vi "AMC_OpenCloseConn.vi"(7 "Open":bool, 8 "error in":errorcluster, 9 "deviceAddress":string="192.168.0.3", 10 "Retry":bool, 11 "ConnID":refnum<k5>) -> (0 "error out":errorcluster, 3 "connection ID":refnum<k5>)   [LabVIEW 2019]
uses:
  <vilib>/Utility/config.llb/Read Key (U32).vi
  <vilib>/Utility/config.llb/Write Key (U32).vi
  <vilib>/Utility/config.llb/Read Key (String).vi
  <vilib>/Utility/config.llb/Read Key (I32).vi
  <vilib>/Utility/config.llb/Read Key (Boolean).vi
  <vilib>/Utility/config.llb/Write Key (String).vi
  <vilib>/Utility/config.llb/Write Key (Boolean).vi
  <vilib>/Utility/config.llb/Write Key (I32).vi
  <vilib>/Utility/config.llb/NI_LVConfig.lvlib
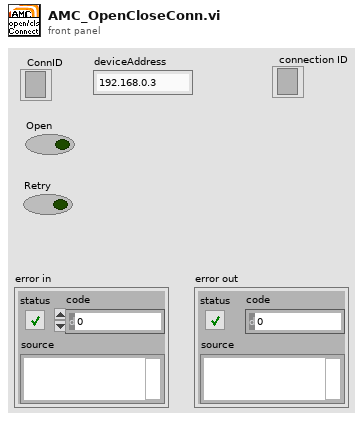
[diagram p1: front panel]
types:
  T1 = enum16{"Répertoire du VI actuel", "Répertoire du parent 1", "Répertoire du parent 2", "Répertoire du parent 3"}
  T2 = typedef "NI_LVConfig.lvlib/Config Data RefNum.ctl" = refnum<k1>
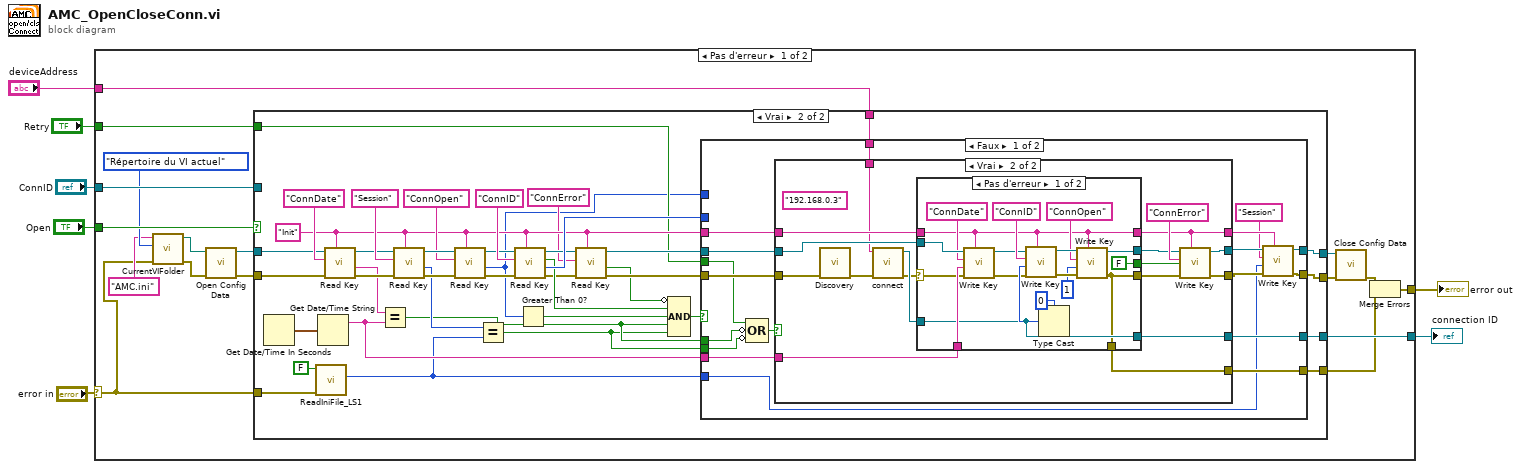
[diagram p0: block diagram]
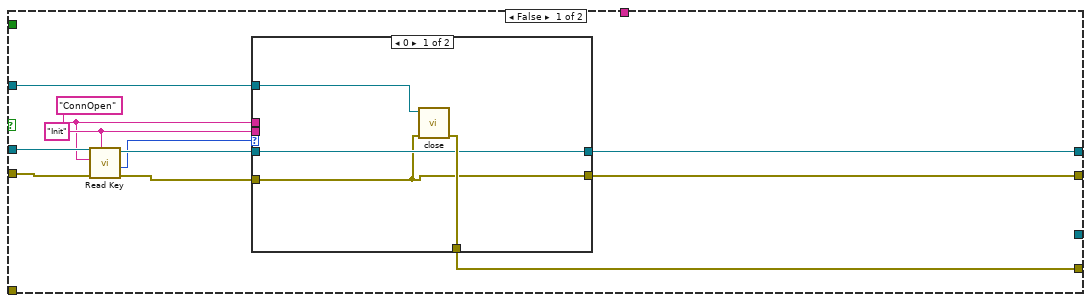
[diagram p2: hidden frame]
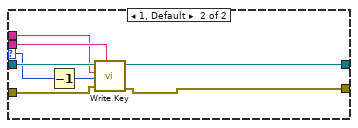
[diagram p3: hidden frame]
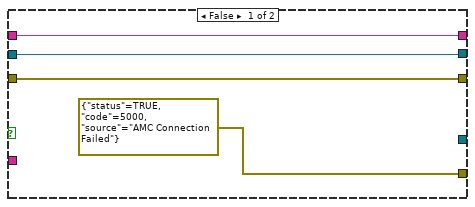
[diagram p4: hidden frame]
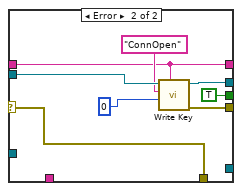
[diagram p5: hidden frame]
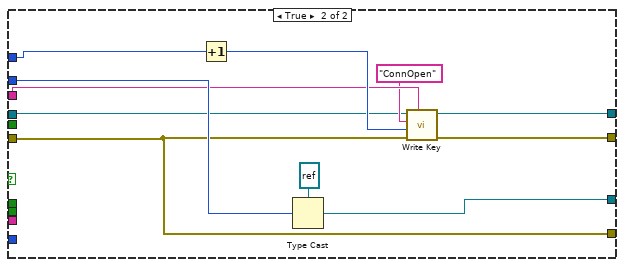
[diagram p6: hidden frame]
diagram:
  n1 = case shown="Pas d'erreur" "error in" {
    selector: "error in" -> [w12 w164]
    tunnel: [w16 w164] -> w7
    tunnel: "Open" -> [w23 _]
    tunnel: [w22 w163] -> w5
    tunnel: "ConnID" -> [w24 w163]
    tunnel: "Retry" -> [w9 _]
    tunnel: "deviceAddress" -> [w8 _]
    frame No Error {
      n2 = call <userlib>:"CurrentVIFolder.vi"("error in (no error)"=w12, "Source"=T1."Répertoire du VI actuel", "NomFichier"="AMC.ini" ("nom ou chemin relatif")) -> ("error out"=w11:errorcluster, "Chemin"=w10:path)  [unwired: 6 in, 1 out]
      n3 = call <vilib>:"Open Config Data.vi"("error in (no error)"=w11, "configuration file path"=w10) -> ("error out"=w21:errorcluster, "refnum"=w20:T2)  [unwired: 7 in, 1 out]
      n4 = case shown="Vrai" w23 {
        tunnel: w24 -> [w34 _]
        tunnel: w12 -> [_ w80]
        tunnel: [_ w76] -> w22
        tunnel: [w33 w71] -> w17
        tunnel: w21 -> [w32 w70]
        tunnel: w20 -> [w29 w69]
        tunnel: [w35 w62] -> w19
        tunnel: [w25 w61] -> w18
        tunnel: w9 -> [_ w51]
        tunnel: w8 -> [_ w48]
        frame False {
          w30 = "Init" ("section")
          w27 = "ConnOpen" ("key")
          n5 = call-poly <vilib>:"Read Key.vi"("section"=w30, "error in (no error)"=w32, "key"=w27, "refnum"=w29) -> ("error out"=w31:errorcluster, "value"=w26:u32, "refnum out"=w28:T2)  [unwired: 4 in, 1 out]
          n6 = case shown="0" w26 {
            selector: w26 -> [_ w40]
            tunnel: [w37 w47] -> w35
            tunnel: w34 -> [w39 _]
            tunnel: [w38 _] -> w33
            tunnel: w31 -> [w36 w46]
            tunnel: w30 -> [_ w45]
            tunnel: w28 -> [w37 w44]
            tunnel: w27 -> [_ w43]
            tunnel: [w36 w42] -> w25
            frame 0 {
              n7 = call <userlib>:"close.vi"("error in"=w36, "connection ID"=w39) -> ("error ECC_connect"=w38:errorcluster)  [unwired: 5 in]
            }
            frame 1, Default {
              n8 = Decrement(x=w40) -> (x-1=w41:u32)
              n9 = call-poly <vilib>:"Write Key.vi"("section"=w45, "error in (no error)"=w46, "value"=w41, "key"=w43, "refnum"=w44) -> ("error out"=w42:errorcluster, "refnum out"=w47:T2)  [unwired: 4 in, 1 out]
            }
          }
        }
        frame True {
          w56 = "Init" ("section")
          n10 = Get Date/Time In Seconds() -> (seconds since 1Jan1904=w79:timestamp)
          n11 = call "ReadIniFile_LS1.vi"("Error in"=w80, "UpdateSess"=FALSE ("IncrSession")) -> ("Session"=w72:i32)  [unwired: 3 in, 6 out]
          n12 = Get Date/Time String(seconds (now)=w79) -> (date string=w73:string)  [unwired: 2 in, 1 out]
          n13 = call-poly <vilib>:"Read Key.vi"("section"=w56, "error in (no error)"=w70, "key"="ConnDate", "refnum"=w69) -> ("error out"=w84:errorcluster, "value"=w78:string, "refnum out"=w82:T2)  [unwired: 4 in, 1 out]
          n14 = Equal?(x=w78, y=w73) -> (x = y?=w55:bool)
          n15 = call-poly <vilib>:"Read Key.vi"("section"=w56, "error in (no error)"=w84, "key"="Session", "refnum"=w82) -> ("error out"=w68:errorcluster, "value"=w67:i32, "refnum out"=w66:T2)  [unwired: 4 in, 1 out]
          n16 = call-poly <vilib>:"Read Key.vi"("section"=w56, "error in (no error)"=w68, "key"="ConnOpen", "refnum"=w66) -> ("error out"=w64:errorcluster, "value"=w49:u32, "refnum out"=w63:T2)  [unwired: 4 in, 1 out]
          n17 = Equal?(x=w67, y=w72) -> (x = y?=w54:bool)
          n18 = call-poly <vilib>:"Read Key.vi"("section"=w56, "error in (no error)"=w64, "key"="ConnID", "refnum"=w63) -> ("error out"=w60:errorcluster, "value"=w77:u32, "found?"=w75:bool, "refnum out"=w57:T2)  [unwired: 4 in]
          n19 = Greater Than 0?(x=w49) -> (x > 0?=w50:bool)
          n20 = call-poly <vilib>:"Read Key.vi"("section"=w56, "error in (no error)"=w60, "key"="ConnError", "refnum"=w57) -> ("error out"=w59:errorcluster, "value"=w52:bool, "refnum out"=w58:T2)  [unwired: 4 in, 1 out]
          n21 = Compound Arithmetic op=AND ("Opérateur arithmétique")(invert w52, w75, w50, w55, w54) -> (w74:bool)
          n22 = case shown="Faux" w74 {
            tunnel: w77 -> [_ w161]
            tunnel: [w100 w160] -> w76
            tunnel: w59 -> [w104 w159]
            tunnel: w58 -> [w103 w153]
            tunnel: w73 -> [w102 _]
            tunnel: w72 -> [w88 _]
            tunnel: w56 -> [w101 w156]
            tunnel: [w99 w159] -> w71
            tunnel: [w90 w152] -> w62
            tunnel: [w89 w154] -> w61
            tunnel: w55 -> [w96 _]
            tunnel: w54 -> [w95 _]
            tunnel: w51 -> [w98 _]
            tunnel: w49 -> [_ w158]
            tunnel: w48 -> [w87 _]
            frame False {
              n23 = Compound Arithmetic op=OR ("Opérateur arithmétique")(w98, invert w96, invert w95) -> (w97:bool)
              n24 = case shown="Vrai" w97 {
                tunnel: w104 -> [w106 w125]
                tunnel: w103 -> [w108 w123]
                tunnel: w102 -> [_ w122]
                tunnel: w101 -> [w105 w121]
                tunnel: [_ w119] -> w100
                tunnel: [w108 w112] -> w94
                tunnel: [w106 w113] -> w93
                tunnel: [errorcluster {"status"=TRUE, "code"=5000, "source"="AMC Connection Failed"} ("error IO") w117] -> w99
                tunnel: [w105 w110] -> w92
                tunnel: w87 -> [_ w109]
                frame False {
                }
                frame True {
                  (unwired) "192.168.0.3" ("deviceAddress")
                  n25 = call <userlib>:"Discovery.vi"("Error In"=w125) -> ("error out"=w124:errorcluster)  [unwired: 9 in, 1 out]
                  n26 = call <userlib>:"connect.vi"("error in"=w124, "deviceAddress"=w109) -> ("error ECC_connect"=w118:errorcluster, "connection ID"=w120:refnum<k5>)  [unwired: 4 in]
                  n27 = case shown="Pas d'erreur" w118 {
                    selector: w118 -> [w136 w145]
                    tunnel: w123 -> [w142 w151]
                    tunnel: w122 -> [w140 _]
                    tunnel: w121 -> [w130 w147]
                    tunnel: w120 -> [w137 _]
                    tunnel: [w137 _] -> w119
                    tunnel: [w131 w150] -> w114
                    tunnel: [w132 w149] -> w115
                    tunnel: [w131 w145] -> w117
                    tunnel: [w130 w147] -> w110
                    tunnel: [FALSE ("value") TRUE ("value")] -> w111
                    frame No Error {
                      n28 = call-poly <vilib>:"Write Key.vi"("section"=w130, "error in (no error)"=w136, "value"=w140, "key"="ConnDate", "refnum"=w142) -> ("error out"=w127:errorcluster, "refnum out"=w128:T2)  [unwired: 4 in, 1 out]
                      n29 = Type Cast(type=u32 0, x=w137) -> (*(type *) &x=w139:u32)
                      n30 = call-poly <vilib>:"Write Key.vi"("section"=w130, "error in (no error)"=w127, "value"=w139, "key"="ConnID", "refnum"=w128) -> ("error out"=w134:errorcluster, "refnum out"=w135:T2)  [unwired: 4 in, 1 out]
                      n31 = call-poly <vilib>:"Write Key.vi"("section"=w130, "error in (no error)"=w134, "value"=u32 1, "key"="ConnOpen", "refnum"=w135) -> ("error out"=w131:errorcluster, "refnum out"=w132:T2)  [unwired: 4 in, 1 out]
                    }
                    frame Error {
                      n32 = call-poly <vilib>:"Write Key.vi"("section"=w147, "value"=u32 0, "key"="ConnOpen", "refnum"=w151) -> ("error out"=w150:errorcluster, "refnum out"=w149:T2)  [unwired: 5 in, 1 out]
                    }
                  }
                  n33 = call-poly <vilib>:"Write Key.vi"("section"=w110, "error in (no error)"=w114, "value"=w111, "key"="ConnError", "refnum"=w115) -> ("error out"=w113:errorcluster, "refnum out"=w112:T2)  [unwired: 4 in, 1 out]
                }
              }
              n34 = call-poly <vilib>:"Write Key.vi"("section"=w92, "error in (no error)"=w93, "value"=w88, "key"="Session", "refnum"=w94) -> ("error out"=w89:errorcluster, "refnum out"=w90:T2)  [unwired: 4 in, 1 out]
            }
            frame True {
              n35 = Increment(x=w158) -> (x+1=w157:u32)
              n36 = Type Cast(type=refnum<k5> refnum ("ConnID"), x=w161) -> (*(type *) &x=w160:refnum<k5>)
              n37 = call-poly <vilib>:"Write Key.vi"("section"=w156, "error in (no error)"=w159, "value"=w157, "key"="ConnOpen", "refnum"=w153) -> ("error out"=w154:errorcluster, "refnum out"=w152:T2)  [unwired: 4 in, 1 out]
            }
          }
        }
      }
      n38 = call <vilib>:"Close Config Data.vi"("error in (no error)"=w18, "refnum"=w19) -> ("error out"=w15:errorcluster)  [unwired: 8 in, 1 out]
      n39 = Merge Errors(w15, w17) -> (w16:errorcluster)
    }
    frame Error {
    }
  }
  "error out" <- w7
  "connection ID" <- w5
